vi "Read Drive Operation.vi"(8 "Command Info":T5) -> (0 "Command Info":T5, 1 "SubSystem Data":T1 {"Auto Path Data"."Commands"."System" items=["FLoating Intake"=2, "Carriage Intake"=1, "Elevator"=0]; "Auto Path Data"."Commands"."System Selection" items=["FLoating Intake"=2, "Carriage Intake"=1, "Elevator"=0]}, 2 "Command Timing":cluster{"Start Time (ms)":u32, "Iterations":i32})   [LabVIEW 2018]
doc: "Returns the details about the currently executing command."
uses:
  <vilib>/Rock Robotics/WPI/Framework/Command Status Info.ctl
  <vilib>/Rock Robotics/WPI/Framework/Completion Status.ctl
  <vilib>/Rock Robotics/WPI/Framework/Completion Notifier.ctl
  Implementation/Drive Setpoints.ctl
  Implementation/Drive Operations.ctl
  Support Code/Path Data.ctl
  Support Code/Availible Command systems for auto.ctl
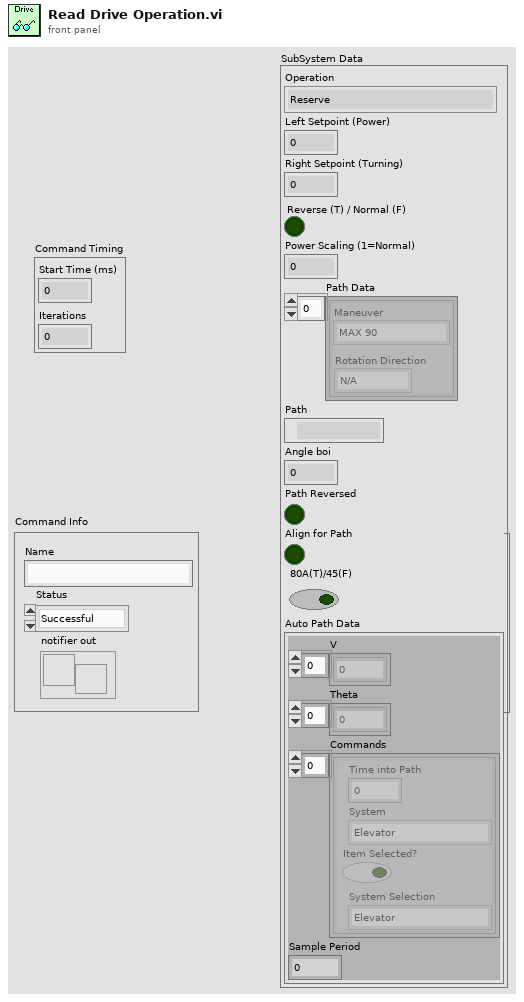
[diagram p1: front panel]
types:
  T1 = typedef "Drive Setpoints.ctl" = cluster{"Operation":T2, "Left Setpoint (Power)":dbl, "Right Setpoint (Turning)":dbl, "Reverse (T) / Normal (F)":bool, "Power Scaling (1=Normal) ":dbl, "Path Data":T3, "Path":path, "Angle boi":dbl, "Path Reversed":bool, "Align for Path":bool, "80A(T)/45(F)":bool, "Auto Path Data":cluster{"V":dbl[], "Theta":dbl[], "Commands":cluster{"Time into Path":dbl, "System":T4, "Item Selected?":bool, "System Selection":T4}[], "Sample Period":dbl}}
  T2 = typedef "Drive Operations.ctl" = enum16{"Reserve", "Read Current", "Immediate", "J-Turn", "Play Back From Log", "Auto-Align"}
  T3 = typedef "Path Data.ctl" = cluster{"Maneuver":enum16{"MAX 90", "MAX 180", "Turn to Home", "Turn to Rocket", "Auto-Align", "Turn to ..."}, "Rotation Direction":enum16{"N/A", "Right", "Left"}}[]
  T4 = typedef "Availible Command systems for auto.ctl" = u16
  T5 = typedef "Command Status Info.ctl" = cluster{"Name":string, "Status":T6, "notifier out":T7}
  T6 = typedef "Completion Status.ctl" = enum16{"Successful", "Aborted", "Incomplete"}
  T7 = typedef "Completion Notifier.ctl" = refnum<notifier>
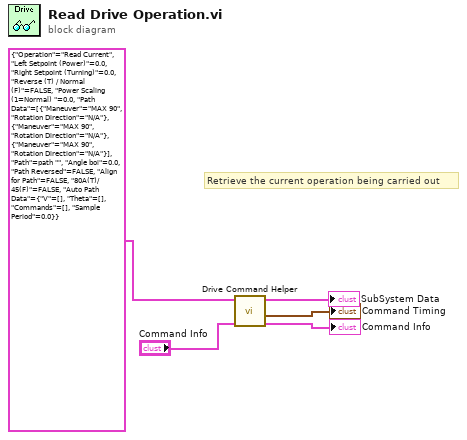
[diagram p0: block diagram]
diagram:
  # "Retrieve the current operation being carried out"
  n1 = call "Drive Command Helper.vi"("Command Info In"="Command Info", "SubSystem Data"=T1 {"Operation"=enum."Read Current", "Left Setpoint (Power)"=0.0, "Right Setpoint (Turning)"=0.0, "Reverse (T) / Normal (F)"=FALSE, "Power Scaling (1=Normal) "=0.0, "Path Data"=[{"Maneuver"=enum."MAX 90", "Rotation Direction"=enum."N/A"}, {"Maneuver"=enum."MAX 90", "Rotation Direction"=enum."N/A"}, {"Maneuver"=enum."MAX 90", "Rotation Direction"=enum."N/A"}], "Path"=path "", "Angle boi"=0.0, "Path Reversed"=FALSE, "Align for Path"=FALSE, "80A(T)/45(F)"=FALSE, "Auto Path Data"={"V"=[], "Theta"=[], "Commands"=[], "Sample Period"=0.0}}) -> ("Command Info Out"=→"Command Info":T5, "Command Timing"=→"Command Timing":cluster{"Start Time (ms)":u32, "Iterations":i32}, "SubSystem Data"=→"SubSystem Data":T1)  [unwired: 7 in]
